vi "AUtoFindTarget.vi"(11 "RobotDriveDevRef":T1) -> ()   [LabVIEW 2015]
uses:
  <vilib>/Rock Robotics/WPI/RobotDrive/WPI_RobotDriveDevRef.ctl
  <vilib>/Rock Robotics/WPI/MotorControl/WPI_MotorControlDeviceRef.ctl
  <vilib>/Rock Robotics/WPI/MotorControl/WPI_MotorControlType.ctl
  <vilib>/Rock Robotics/SystemInterfaces/DIO/FPGA_DIOPWMChannel.ctl
  <vilib>/Rock Robotics/WPI/PWM/WPI_PWMDeadband.ctl
  <vilib>/Rock Robotics/WPI/CAN/Jaguar/SubVIs/WPI_CANJaguar_ControlMode.ctl
  <vilib>/Rock Robotics/WPI/CAN/TalonSRX/WPI_CANTalonSRX_APIControlMode.ctl
  <vilib>/Rock Robotics/Network Tables/NT Read Number.vi
  Robot Global Data.vi
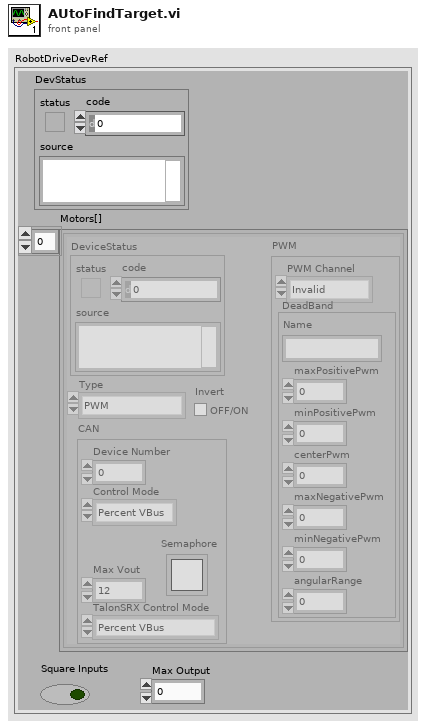
[diagram p1: front panel]
types:
  T1 = typedef "WPI_RobotDriveDevRef.ctl" = cluster{"DevStatus":errorcluster, "Motors[]":T2[], "Square Inputs":bool, "Max Output":dbl}
  T2 = typedef "WPI_MotorControlDeviceRef.ctl" = cluster{"DeviceStatus":errorcluster, "Type":T3, "PWM":cluster{"PWM Channel":T4, "DeadBand":T5}, "CAN":cluster{"Device Number":u8, "Control Mode":T6, "Semaphore":T7, "Max Vout":dbl, "TalonSRX Control Mode":T8}, "Invert":bool}
  T3 = typedef "WPI_MotorControlType.ctl" = enum16{"PWM", "CAN", "CANTalonSRX"}
  T4 = typedef "FPGA_DIOPWMChannel.ctl" = enum8{"PWM 0", "PWM 1", "PWM 2", "PWM 3", "PWM 4", "PWM 5", "PWM 6", "PWM 7", "PWM 8", "PWM 9", "PWM MXP 0", "PWM MXP 1", "PWM MXP 2", "PWM MXP 3", "PWM MXP 4", "PWM MXP 5", "PWM MXP 6", "PWM MXP 7", "PWM MXP 8", "PWM MXP 9", "Invalid"}
  T5 = typedef "WPI_PWMDeadband.ctl" = cluster{"Name":string, "maxPositivePwm":i32, "minPositivePwm":i32, "centerPwm":i32, "maxNegativePwm":i32, "minNegativePwm":i32, "angularRange":u16}
  T6 = typedef "WPI_CANJaguar_ControlMode.ctl" = enum8{"Percent VBus", "Current", "Speed", "Position", "Voltage"}
  T7 = typedef "Semaphore RefNum" = refnum<k1>
  T8 = typedef "WPI_CANTalonSRX_APIControlMode.ctl" = enum8{"Percent VBus", "Speed", "Position", "Slave", "Unchanged / Invalid", "Voltage Compensation", "Current", "Motion Profile"}
  T9 = cluster{"Distance (ft)":dbl, "Center":cluster{dbl, dbl}, "Normalized Rect":cluster{"Numeric":dbl, "Numeric 2":dbl, "Numeric 3":dbl, "Numeric 5":dbl}}[]
  T10 = cluster{"Distance (ft)":dbl, "Center":cluster{dbl, dbl}, "Normalized Rect":cluster{"Numeric":dbl, "Numeric 2":dbl, "Numeric 3":dbl, "Numeric 5":dbl}}
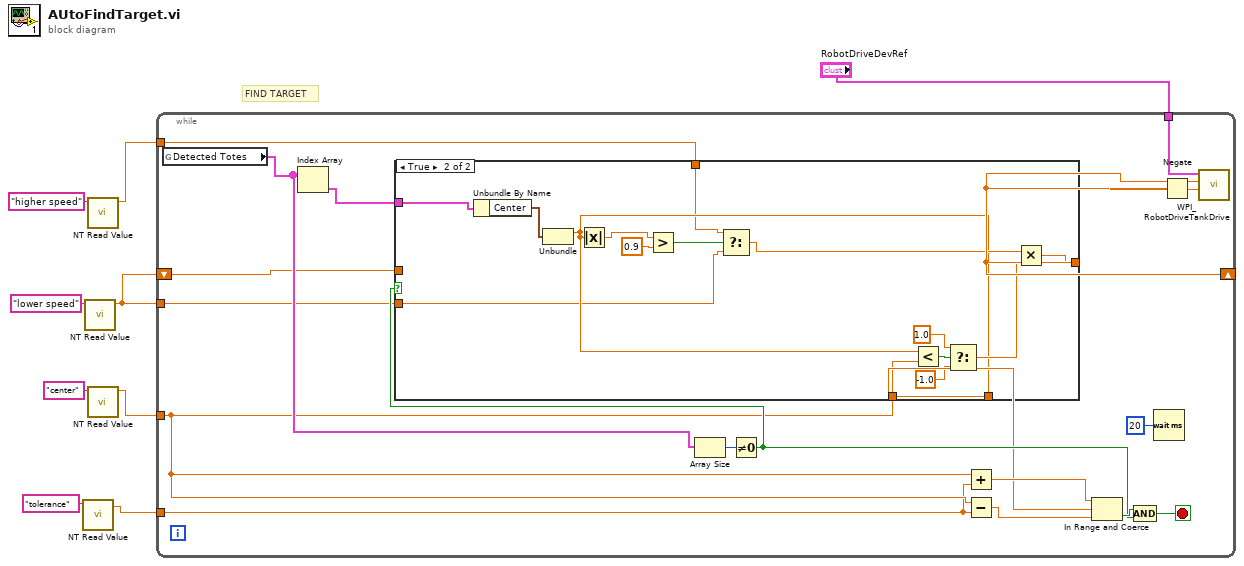
[diagram p0: block diagram]
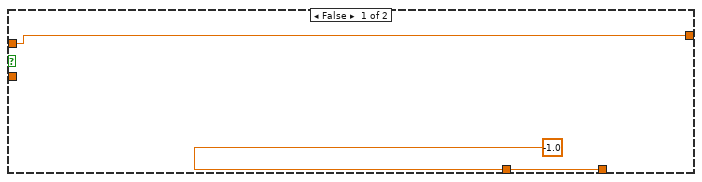
[diagram p2: hidden frame]
diagram:
  # "FIND TARGET"
  n1 = call-poly <vilib>:"NT Read Value.vi"("Name"="tolerance") -> ("Numeric"=w9:dbl)  [unwired: 9 in, 1 out]
  n2 = call-poly <vilib>:"NT Read Value.vi"("Name"="lower speed") -> ("Numeric"=w3:dbl)  [unwired: 9 in, 1 out]
  n3 = call-poly <vilib>:"NT Read Value.vi"("Name"="higher speed") -> ("Numeric"=w5:dbl)  [unwired: 9 in, 1 out]
  n4 = call-poly <vilib>:"NT Read Value.vi"("Name"="center") -> ("Numeric"=w7:dbl)  [unwired: 9 in, 1 out]
  n5 = while {
    tunnel: "RobotDriveDevRef" -> [w25]
    shift-right: [w15] -> _
    shift-left: w3 -> [w16]
    tunnel: w3 -> [w13]
    tunnel: w5 -> [w12]
    tunnel: w7 -> [w11]
    tunnel: w9 -> [w10]
    stop <- w24 stop-if-true
    n6 = global read "Robot Global Data.vi" "Detected Totes"() -> (w23:T9)
    n7 = Index Array(array=w23) -> (element=w27:T10)  [unwired: 1 in]
    n8 = Array Size(array=w23) -> (size(s)=w22:i32)
    n9 = Not Equal To 0?(x=w22) -> (x != 0?=w17:bool)
    n10 = case shown="True" w17 {
      tunnel: w27 -> [_ w44]
      tunnel: w11 -> [_ w42]
      tunnel: [w29 w33] -> w15
      tunnel: w16 -> [w29 _]
      tunnel: [-1.0 ("x") w32] -> w14
      tunnel: w13 -> [_ w31]
      tunnel: w12 -> [_ w30]
      frame False {
      }
      frame True {
        n11 = Unbundle By Name(w44) -> ("Center"=w43:cluster{dbl, dbl})
        n12 = Unbundle(w43) -> (w32:dbl)  [unwired: 1 out]
        n13 = Absolute Value(x=w32) -> (abs(x)=w41:dbl)
        n14 = Greater?(x=w41, y=0.9) -> (0:w39:bool)
        n15 = Select(t=w30, s=w39, f=w31) -> (s? t:f=w35:dbl)
        n16 = Less?(x=w32, y=w42) -> (x < y?=w38:bool)
        n17 = Select(t=1.0, s=w38, f=-1.0) -> (s? t:f=w34:dbl)
        n18 = Multiply(x=w35, y=w34) -> (x*y=w33:dbl)
      }
    }
    n19 = Add(x=w11, y=w10) -> (x+y=w19:dbl)
    n20 = Subtract(x=w11, y=w10) -> (x-y=w18:dbl)
    n21 = In Range and Coerce(upper limit=w19, x=w14, lower limit=w18) -> (In Range?=w26:bool)  [unwired: 1 out]
    n22 = Compound Arithmetic op=AND(w26, w17) -> (w24:bool)
    n23 = Wait (ms)(milliseconds to wait=u32 20) -> ()  [unwired: 1 out]
    n24 = Negate(x=w15) -> (-x=w20:dbl)
    n25 = call <vilib>:"WPI_RobotDriveTankDrive.vi"("Right axis value"=w20, "Left axis value"=w15, "RobotDriveDevRef"=w25) -> ()  [unwired: 6 in, 3 out]
  }
